vi "Get Value for package_template_enum.vi"(8 "error in (no error)":errorcluster, 11 "gRPC ID":T1) -> (0 "error out":errorcluster, 2 "value in proto":u32, 3 "gRPC ID Out":T1)   [LabVIEW 2019, in "Service Template.lvlib"]
uses:
  Service Template.lvlib
  <vilib>/gRPC/LabVIEW gRPC Library/Shared/grpcId.ctl
  gRPC Scripting Tools/gRPC Template Creation Utility.lvlib
  <vilib>/gRPC/LabVIEW gRPC Library/grpc-lvsupport-release.lvlib
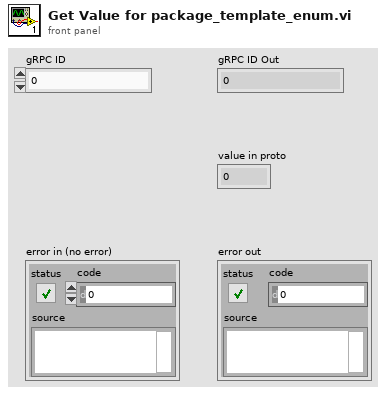
[diagram p1: front panel]
types:
  T1 = typedef "grpc-lvsupport-release.lvlib/grpcId.ctl" = u64
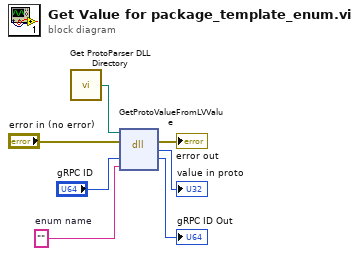
[diagram p0: block diagram]
diagram:
  w6 = ""  # enum name
  n1 = call "Get ProtoParser DLL Directory.vi"() -> ("Proto Parser Directory"=w7:path)
  n2 = dll-call lib="C:/Source/grpc-labview/build/Debug/labview_grpc_server.dll" fn="GetProtoValueFromLVValue"(path in=w7, error in="error in (no error)", "gRPC ID in"="gRPC ID", "enum name"=w6) -> (error out=→"error out":errorcluster, "value in proto"=→"value in proto":u32, "gRPC ID in"=→"gRPC ID Out":u64)  [unwired: 2 in, 1 out]
